vi "Voltage (non-regeneration) - Continuous Output.vi"() -> ()   [LabVIEW 2012]
doc: "This example demonstrates how to continuously generate an analog output waveform by providing new data to the output buffer as the task is running.\n\nThis example is useful if you want to generate a non-repeating waveform, make updates on-the-fly, or generate a frequency that is not an even divide-down of your sample clock."
uses:
  <vilib>/DAQmx/write.llb/DAQmx Write (Analog 1D Wfm NChan NSamp).vi
  <vilib>/DAQmx/create/channels.llb/DAQmx Create Channel (AO-Voltage-Basic).vi
  <vilib>/DAQmx/configure/timing.llb/DAQmx Timing (Sample Clock).vi
  <vilib>/DAQmx/miscellaneous.llb/DAQmx Fill In Error Info.vi
  <resource>/objmgr/daqmx.rc
  <vilib>/measure/NI_MABase.lvlib
panel:
  in  "Output Array":T1(array[cluster])=[{"Waveform Type"=0, "Amplitude"=1.0, "Frequency"=10.0}] {"Frequency" format="%0.2p"; "Amplitude" format="%0.2p"; "Waveform Type" items=["Sine Wave", "Triangle Wave", "Square Wave", "Sawtooth Wave"]}
  in  "Number of Samples":i32=1000
  in  "Stop":bool
  out "Waveform Graph":waveform(dbl)[](graph)=[{"t0"=timestamp(0 s since 1904-01-01), "dt"=0.001, "Y"=[]}]
  in  "Sample Rate":dbl=1000.0
  in  "Sample Clock Source":tag="OnboardClock"
  in  "Max Voltage":dbl=5.0
  in  "Min Voltage":dbl=-5.0
  in  "Physical Channel(s)":tag="Dev1/ao0"
  out "Actual Sample Rate":dbl=1000.0 format="%0.2f"
  # "Channel Settings"
  # "Output"
  # "Timing and Buffer Settings"
  # "Waveform Settings"
  # "The number of elements in the waveform array\nmust equal the number of channels in the task."
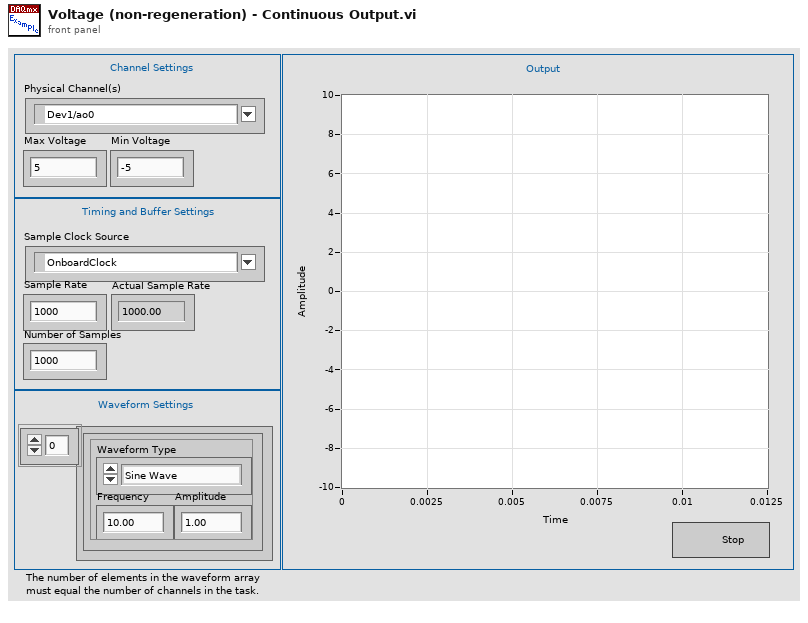
[diagram p1: front panel]
types:
  T1 = cluster{"Waveform Type":u16, "Amplitude":dbl, "Frequency":dbl}[]
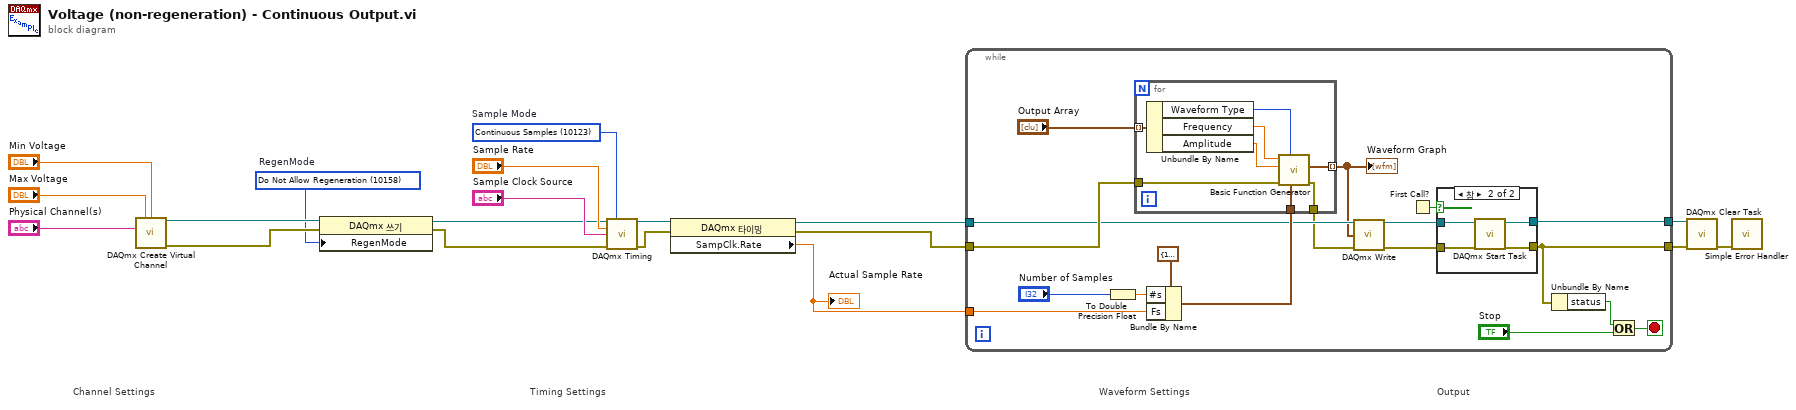
[diagram p0: block diagram]
diagram:
  w7 = 10158 items=["Allow Regeneration"=10097, "Do Not Allow Regeneration"=10158]  # RegenMode
  w17 = 10123 items=["Finite Samples"=10178, "Continuous Samples"=10123, "Hardware Timed Single Point"=12522]  # Sample Mode
  # "Output"
  # "Waveform Settings"
  # "Timing Settings"
  # "Channel Settings"
  n1 = call-poly <vilib>:"DAQmx Create Virtual Channel.vi"("maximum value"="Max Voltage", "minimum value"="Min Voltage", "physical channels"="Physical Channel(s)") -> ("task out"=w9:refnum<k21>, "error out"=w8:errorcluster)  [unwired: 11 in]
  n2 = property class="DAQmx 쓰기"(reference=w9, error in=w8, "RegenMode"=w7) -> (reference out=w5:refnum<k21>, error out=w6:errorcluster)
  n3 = call-poly <vilib>:"DAQmx Timing.vi"("task/channels in"=w5, "sample mode"=w17, "rate"="Sample Rate", "source"="Sample Clock Source", "error in"=w6) -> ("task out"=w19:refnum<k21>, "error out"=w18:errorcluster)  [unwired: 9 in]
  n4 = property class="DAQmx 타이밍"(reference=w19, error in=w18) -> (reference out=w2:refnum<k21>, error out=w1:errorcluster, "SampClk.Rate"=w10:dbl)
  "Actual Sample Rate" <- w10
  n5 = while {
    tunnel: w1 -> [w37]
    tunnel: w10 -> [w35]
    tunnel: w2 -> [w33]
    tunnel: [w24] -> w4
    tunnel: [w23] -> w3
    stop <- w21 stop-if-true
    n6 = To Double Precision Float(number="Number of Samples") -> (double precision float=w27:dbl)
    n7 = Bundle By Name(cluster=cluster{"Fs":dbl, "#s":dbl} {"Fs"=1000.0, "#s"=1000.0} ("sampling info"), "#s"=w27, "Fs"=w35) -> (w34:cluster{"Fs":dbl, "#s":dbl})
    n8 = for {
      tunnel: w37 -> [w51]
      tunnel: w34 -> [w50]
      tunnel: [w49] -> w30
      tunnel: "Output Array" -> [w48] mode=indexing
      tunnel: [w44] -> w28 mode=indexing
      n9 = Unbundle By Name(w48) -> ("Waveform Type"=w47:u16, "Frequency"=w46:dbl, "Amplitude"=w45:dbl)
      n10 = call <vilib>:"Basic Function Generator.vi"("sampling info"=w50, "signal type"=w47, "error in (no error)"=w51, "amplitude"=w45, "frequency"=w46) -> ("error out"=w49:errorcluster, "signal out"=w44:waveform(dbl))  [unwired: 4 in, 1 out]
    }
    "Waveform Graph" <- w28
    n11 = call-poly <vilib>:"DAQmx Write.vi"("task/channels in"=w33, "data"=w28, "error in"=w30) -> ("task out"=w32:refnum<k21>, "error out"=w31:errorcluster)  [unwired: 10 in, 1 out]
    n12 = First Call?() -> (First Call?: T/F=w25:bool)
    n13 = case shown="참" w25 {
      tunnel: w32 -> [w38 w43]
      tunnel: w31 -> [w39 w42]
      tunnel: [w38 w41] -> w24
      tunnel: [w39 w40] -> w23
      frame False {
      }
      frame True {
        n14 = call <vilib>:"DAQmx Start Task.vi"("task/channels in"=w43, "error in"=w42) -> ("task out"=w41:refnum<k21>, "error out"=w40:errorcluster)  [unwired: 12 in]
      }
    }
    n15 = Unbundle By Name(w23) -> ("status"=w20:bool)
    n16 = Or(x=w20, y="Stop") -> (x .or. y?=w21:bool)
  }
  n17 = call <vilib>:"DAQmx Clear Task.vi"("task in"=w4, "error in"=w3) -> ("error out"=w16:errorcluster)  [unwired: 13 in]
  n18 = call <vilib>:"Simple Error Handler.vi"("error in (no error)"=w16) -> ()  [unwired: 4 in, 5 out]
